vi "Challenge Cipher.vi"(11 "Challenge":string) -> (3 "Response":string)   [LabVIEW 2018, in "Telnet V2.lvlib" / "Telnet V2.lvclass"]
doc: "This is the Cipher that receives the Challenge Message and processes it to return the appropriate Key Response. \n\nThis VI is proprietary to Lumiar and is not to be distributed outside of Luminar Tech."
uses:
  Telnet V2.lvclass
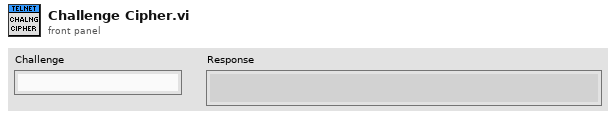
[diagram p1: front panel]
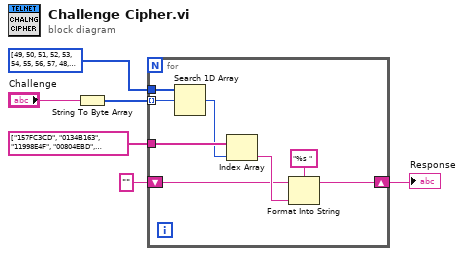
[diagram p0: block diagram]
diagram:
  n1 = String To Byte Array(string="Challenge") -> (unsigned byte array=w4:u8[])
  n2 = for {
    tunnel: u8[] [49, 50, 51, 52, 53, 54, 55, 56, 57, 48, 113, 119, 101, 114, 116, 121, 117, 105, 111, 112, 97, 115, 100, 102, 103, 104, 106, 107, 108, 122, 120, 99, 118, 98, 110, 109, 81, 87, 69, 82, 84, 89, 85, 73, 79, 80, 65, 83, 68, 70, 71, 72, 74, 75, 76, 90, 88, 67, 86, 66, 78, 77, 45, 61, 95, 43] ("Challenge Cipher") -> [w14]
    tunnel: w4 -> [w13] mode=indexing
    tunnel: string[] ["157FC3CD", "0134B163", "11998E4F", "00804EBD", "1590D80E", "17A9786D", "0E833F5C", "1469A357", "04698844", "0EC8636F", "10F93824", "117AF4FF", "180C480E", "0234AD15", "029104F8", "04C2E5BB", "1141350D", "11727FF9", "113BC818", "0937CEB0", "068AB594", "0EE4170E", "143F61AD", "0E9F903B", "0FCAFAC3", "11DDDE9F", "104C14FB", "0000EE83", "056AF033", "0B045F60", "068A5178", "0FAF9CEB", "038B036C", "1556B7C7", "0FEC7A8E", "0D6D34D2", "15251917", "0BDCD8F0", "0FDE2660", "088A853B", "054FDD9A", "10484921", "19FFFC40", "11AEE2BC", "182D7F2F", "044618EA", "02D77C1D", "17B85C86", "010C7FE3", "0E47969F", "04FAA912", "0430B36B", "0BD5A6A3", "19B5C039", "11FB1063", "15EA90A2", "1201FF09", "1001B123", "1756AC31", "0F93292C", "0E635F00", "1A142EA0", "0FF47F0B", "1AD2209B", "09BAC4ED", "1AEB7A7F"] ("Mapped Word") -> [w12]
    shift-right: [w7] -> w1
    shift-left: "" -> [w8]
    n3 = Search 1D Array(1D array=w14, element=w13) -> (index of element=w11:i32)  [unwired: 1 in]
    n4 = Index Array(array=w12, index=w11) -> (element=w9:string)
    n5 = Format Into String(format string="%s ", initial string=w8, w9) -> (resulting string=w7:string)  [unwired: 1 in, 1 out]
  }
  "Response" <- w1
